vi "Коши.vi"() -> ()   [LabVIEW 2018]
uses:
  <vilib>/gmath/NI_Gmath.lvlib
panel:
  in  "angle":dbl=210.0
  in  "V":dbl=0.42
  out "Ep":dbl=0.13046191956905975
  out "Ek":dbl=0.08819999999999999
  in  "h (step rate)":dbl=0.1 format="%#_13g"
  out "sum 2":dbl=530.0
  out "sum":dbl=428.4469162488062
  in  "method":enum16{"Эйлер", "Рунге-Кутта"}(ring)
  in  "Planet #2":cluster{"x":dbl, "y":dbl}={"x"=-23.0, "y"=14.0}
  in  "Planet #1":cluster{"x":dbl, "y":dbl}={"x"=6.0, "y"=5.0}
  in  "y0":dbl=-4.0
  in  "x0":dbl=1.0
  out "XY Graph":T1(graph)=[{"X Values (solution)"=[6.0], "X Values (solution)"=[5.0]}, {"X Values (solution)"=[-23.0], "X Values (solution)"=[14.0]}, {"X Values (solution)"=array[30015 elements], "X Values (solution)"=array[30015 elements]}, {"X Values (solution)"=[1.0], "X Values (solution)"=[-4.0]}]
  in  "time end":dbl=3001.4 format="%.2f"
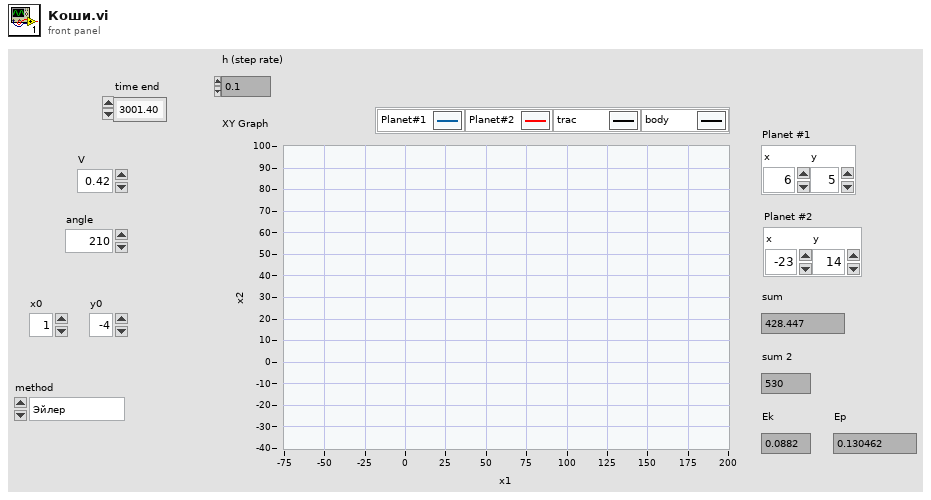
[diagram p1: front panel]
types:
  T1 = cluster{"X Values (solution)":dbl[], "X Values (solution)":dbl[]}[]
  T2 = cluster{"X Values (solution)":dbl[], "X Values (solution)":dbl[]}
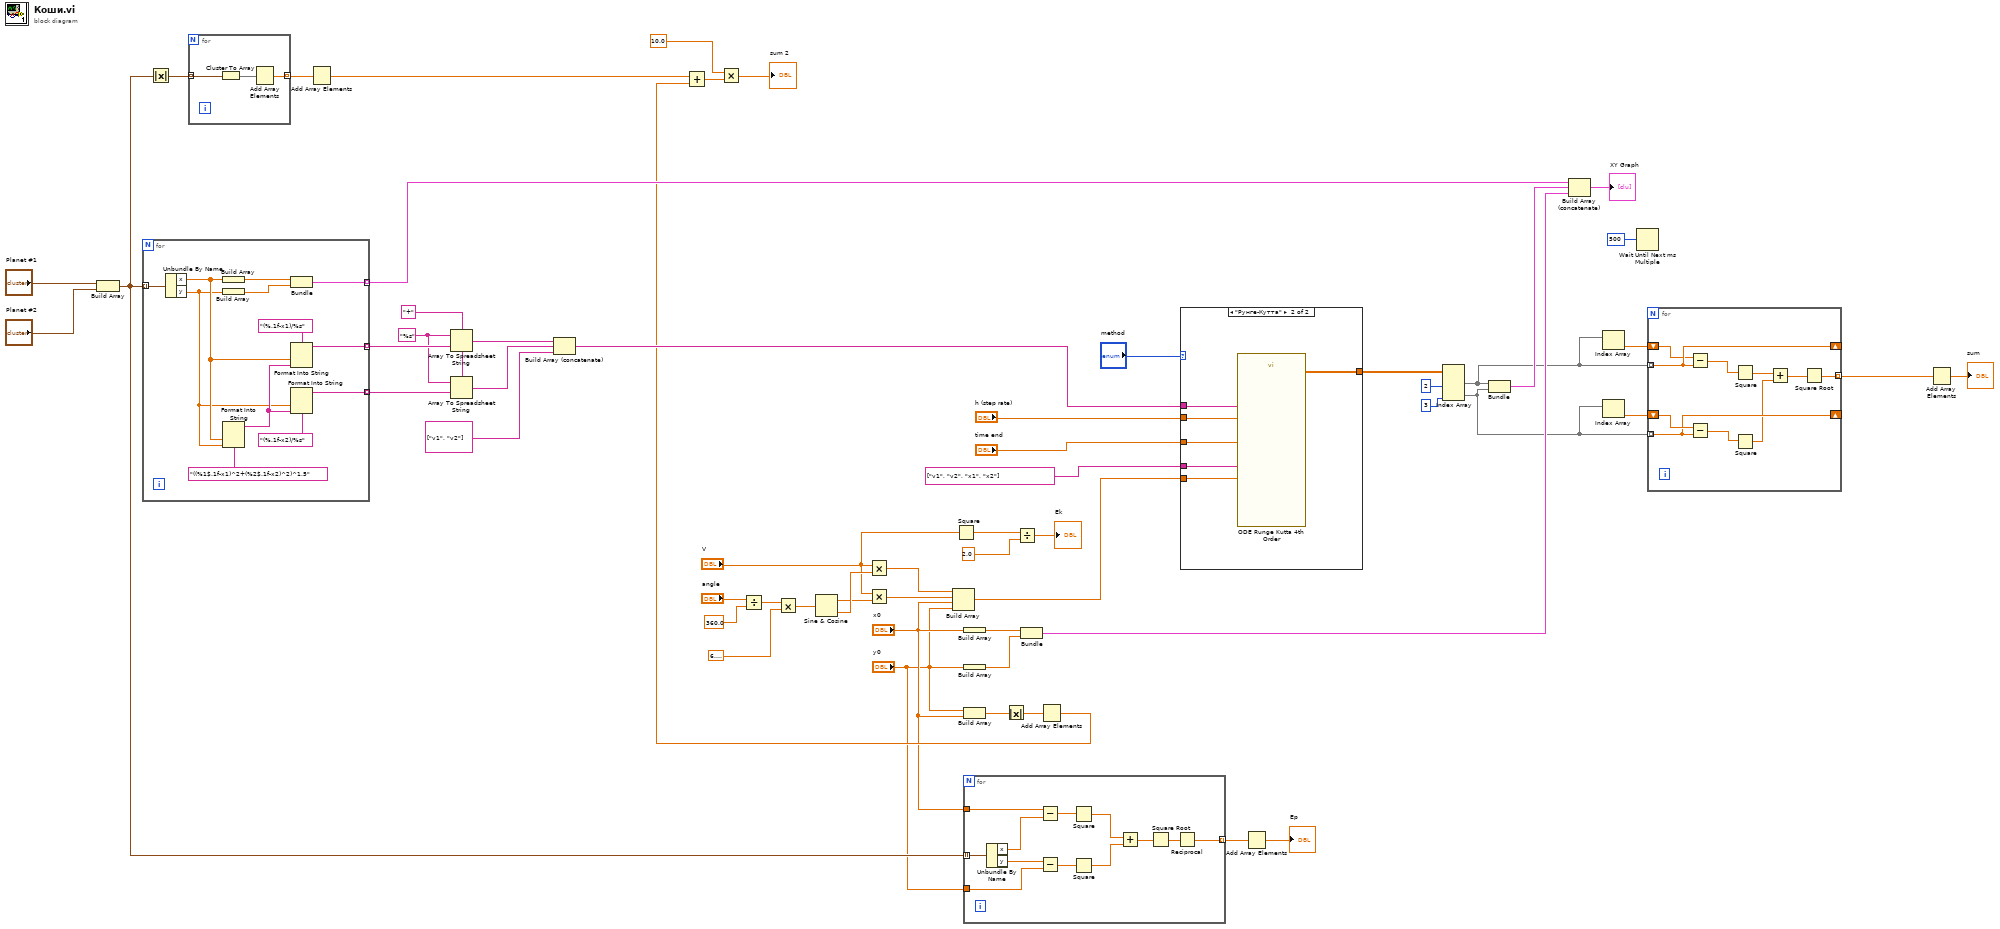
[diagram p0: block diagram]
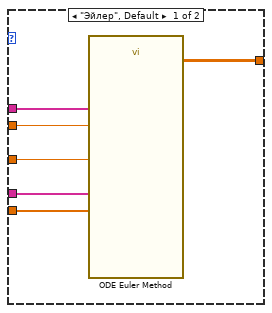
[diagram p2: hidden frame]
diagram:
  w38 = "+" ("delimiter (Tab)")
  w39 = "%s" ("format string")
  n1 = Build Array("Planet #1", "Planet #2") -> (w18:cluster{"x":dbl, "y":dbl}[])
  n2 = for {
    tunnel: w18 -> [w68] mode=indexing
    tunnel: [w62] -> w35 mode=indexing
    tunnel: [w61] -> w41 mode=indexing
    tunnel: [w60] -> w40 mode=indexing
    n3 = Unbundle By Name(w68) -> ("x"=w66:dbl, "y"=w64:dbl)
    n4 = Build Array(w66) -> (w70:dbl[])
    n5 = Build Array(w64) -> (w69:dbl[])
    n6 = Format Into String(format string="((%1$.1f-x1)^2+(%2$.1f-x2)^2)^1,5", w66, w64) -> (resulting string=w65:string)  [unwired: 2 in, 1 out]
    n7 = Bundle(w70, w69) -> (w62:cluster{dbl[], dbl[]})  [unwired: 1 in]
    n8 = Format Into String(format string="(%.1f-x1)/%s", w66, w65) -> (resulting string=w61:string)  [unwired: 2 in, 1 out]
    n9 = Format Into String(format string="(%.1f-x2)/%s", w64, w65) -> (resulting string=w60:string)  [unwired: 2 in, 1 out]
  }
  n10 = Absolute Value(x=w18) -> (abs(x)=w27:cluster{"x":dbl, "y":dbl}[])
  n11 = for {
    tunnel: w27 -> [w73] mode=indexing
    tunnel: [w71] -> w26 mode=indexing
    n12 = Cluster To Array(cluster=w73) -> (array=w72:dbl[])
    n13 = Add Array Elements(numeric array=w72) -> (sum=w71:dbl)
  }
  n14 = Add Array Elements(numeric array=w26) -> (sum=w22:dbl)
  n15 = Array To Spreadsheet String(delimiter (Tab)=w38, array=w41, 3:w39) -> (spreadsheet string=w37:string)
  n16 = Array To Spreadsheet String(delimiter (Tab)=w38, array=w40, 3:w39) -> (spreadsheet string=w36:string)
  n17 = Build Array (concatenate)(w37, w36, string[] ["v1", "v2"] ("F(X,t) (right sides of the ODE\nas functions of X and t)")) -> (w48:string[])
  n18 = Divide(x="angle", y=360.0) -> (x/y=w8:dbl)
  n19 = Multiply(x=w8, y=6.283185307179586) -> (x*y=w9:dbl)
  n20 = Sine & Cosine(0:w9) -> (1:w5:dbl, 2:w6:dbl)
  n21 = Multiply(x="V", y=w6) -> (x*y=w3:dbl)
  n22 = Multiply(x="V", y=w5) -> (x*y=w4:dbl)
  n23 = Build Array(w3, w4, "x0", "y0") -> (w47:dbl[])
  n24 = Square(x="V") -> (x^2=w1:dbl)
  n25 = Build Array("x0") -> (w46:dbl[])
  n26 = Build Array("y0") -> (w45:dbl[])
  n27 = Build Array("y0", "x0") -> (w25:dbl[])
  n28 = for {
    tunnel: w18 -> [w85] mode=indexing
    tunnel: "x0" -> [w84]
    tunnel: "y0" -> [w81]
    tunnel: [w74] -> w15 mode=indexing
    n29 = Unbundle By Name(w85) -> ("x"=w83:dbl, "y"=w82:dbl)
    n30 = Subtract(x=w84, y=w83) -> (x-y=w80:dbl)
    n31 = Subtract(x=w82, y=w81) -> (x-y=w79:dbl)
    n32 = Square(x=w80) -> (x^2=w78:dbl)
    n33 = Square(x=w79) -> (x^2=w77:dbl)
    n34 = Add(x=w78, y=w77) -> (x+y=w76:dbl)
    n35 = Square Root(x=w76) -> (sqrt(x)=w75:dbl)
    n36 = Reciprocal(x=w75) -> (1/x=w74:dbl)
  }
  n37 = Absolute Value(x=w25) -> (abs(x)=w24:dbl[])
  n38 = Divide(x=w1, y=2.0) -> (x/y=→"Ek":dbl)
  n39 = Bundle(w46, w45) -> (w44:cluster{dbl[], dbl[]})  [unwired: 1 in]
  n40 = Add Array Elements(numeric array=w24) -> (sum=w23:dbl)
  n41 = Add(x=w22, y=w23) -> (x+y=w21:dbl)
  n42 = Multiply(x=10.0, y=w21) -> (x*y=→"sum 2":dbl)
  n43 = case shown="\"Рунге-Кутта\"" "method" {
    tunnel: "h (step rate)" -> [w91 w97]
    tunnel: "time end" -> [w90 w96]
    tunnel: string[] ["v1", "v2", "x1", "x2"] ("X (name of variables)") -> [w89 w95]
    tunnel: [w88 w94] -> w55
    tunnel: w48 -> [w87 w93]
    tunnel: w47 -> [w86 w92]
    frame "Эйлер", Default {
      n44 = call <vilib>:"ODE Euler Method.vi"("time end"=w90, "h (step rate)"=w91, "X0"=w86, "X (name of variables)"=w89, "F(X,t) (right sides of the ODE\nas functions of X and t)"=w87) -> ("X Values (solution)"=w88:dbl[][])  [unwired: 2 in, 3 out]
    }
    frame "Рунге-Кутта" {
      n45 = call <vilib>:"ODE Runge Kutta 4th Order.vi"("time end"=w96, "h (step rate)"=w97, "X0"=w92, "X (name of variables)"=w95, "F(X,t) (right sides of the ODE\nas functions of X and t)"=w93) -> ("X Values (solution)"=w94:dbl[][])  [unwired: 2 in, 3 out]
    }
  }
  n46 = Add Array Elements(numeric array=w15) -> (sum=→"Ep":dbl)
  n47 = Index Array(array=w55, index (col) #1=2 ("disabled index (col)"), index (col) #2=3 ("index (col)")) -> (element #1=w33:dbl[], element #2=w31:dbl[])  [unwired: 2 in]
  n48 = Bundle("X Values (solution)"=w33, "X Values (solution)"=w31) -> (w51:T2)  [unwired: 1 in]
  n49 = Build Array (concatenate)(w35, w51, w44) -> (→"XY Graph":T1)
  n50 = Index Array(array=w33) -> (element=w32:dbl)  [unwired: 1 in]
  n51 = Index Array(array=w31) -> (element=w30:dbl)  [unwired: 1 in]
  n52 = Wait Until Next ms Multiple(millisecond multiple=u32 500) -> ()  [unwired: 1 out]
  n53 = for {
    tunnel: w33 -> [w107] mode=indexing
    shift-right: [w107] -> _
    shift-left: w32 -> [w106]
    tunnel: w31 -> [w104] mode=indexing
    shift-right: [w104] -> _
    shift-left: w30 -> [w105]
    tunnel: [w98] -> w29 mode=indexing
    n54 = Subtract(x=w106, y=w107) -> (x-y=w103:dbl)
    n55 = Subtract(x=w105, y=w104) -> (x-y=w102:dbl)
    n56 = Square(x=w103) -> (x^2=w101:dbl)
    n57 = Square(x=w102) -> (x^2=w100:dbl)
    n58 = Add(x=w101, y=w100) -> (x+y=w99:dbl)
    n59 = Square Root(x=w99) -> (sqrt(x)=w98:dbl)
  }
  n60 = Add Array Elements(numeric array=w29) -> (sum=→"sum":dbl)
